vi "phy_packet_decoder.vi"(11 "bits":u8[](array[numeric])) -> (3 "string Array":string[](array[string]))   [LabVIEW 2014]
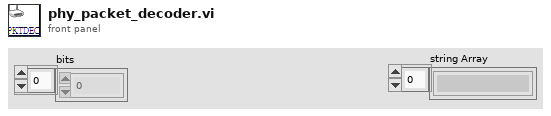
[diagram p1: front panel]
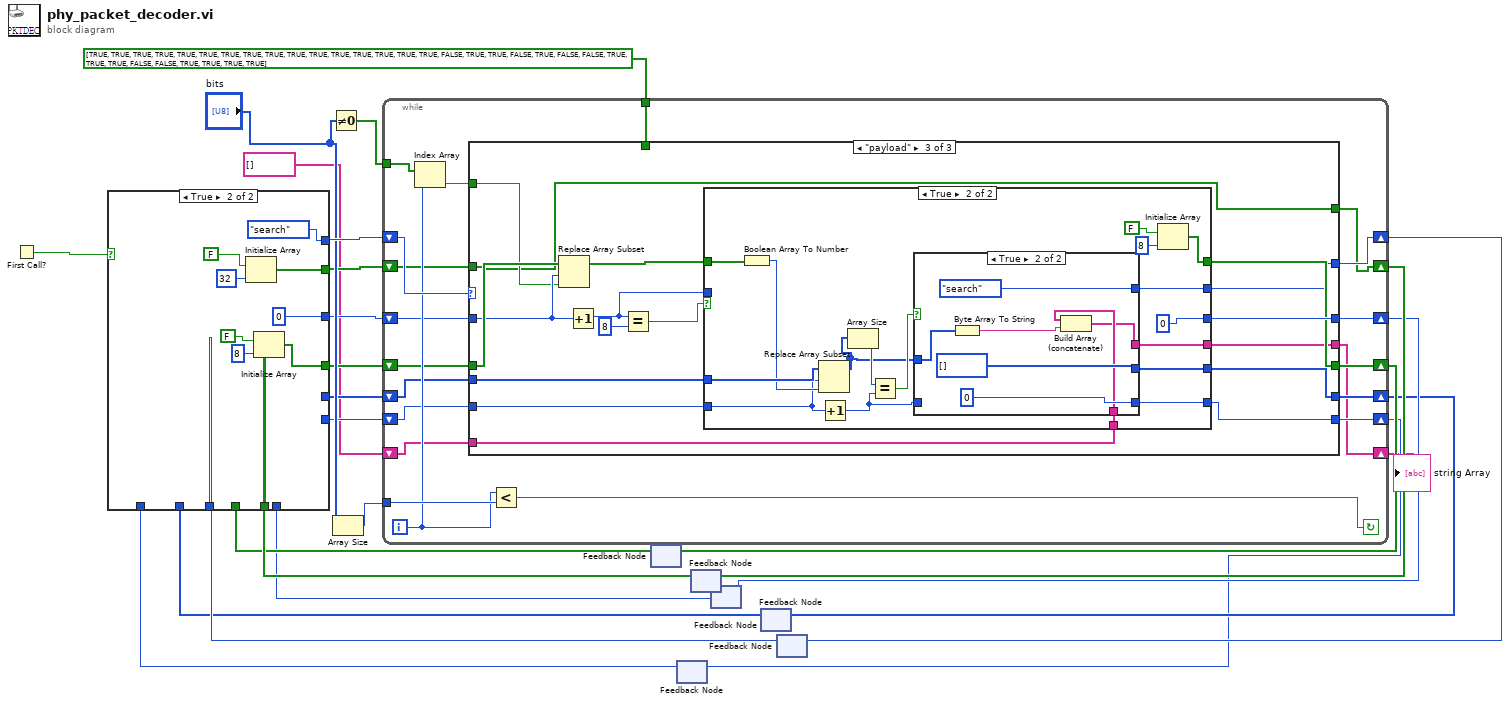
[diagram p0: block diagram]
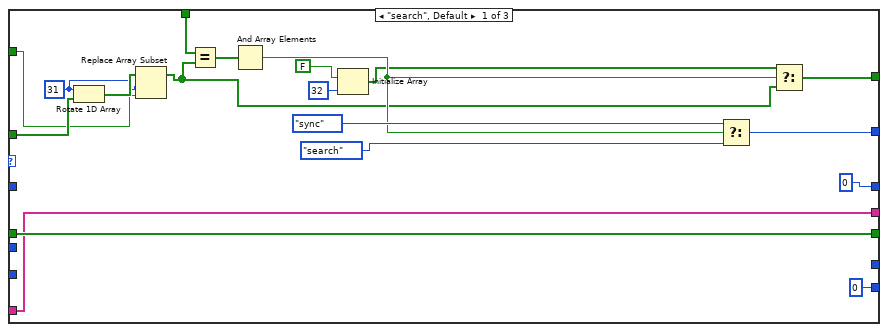
[diagram p3: hidden frame]
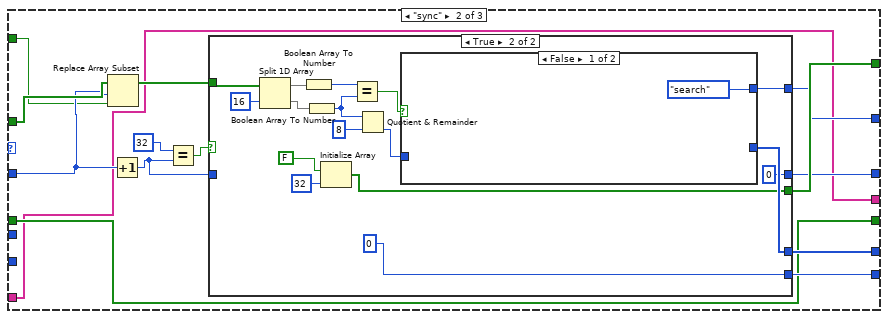
[diagram p4: hidden frame]
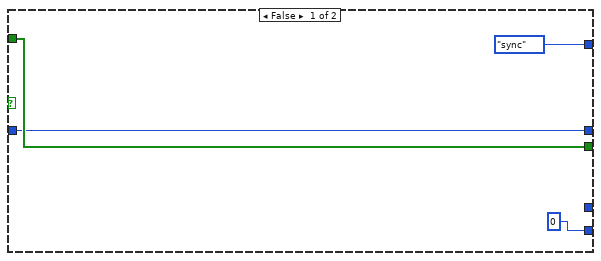
[diagram p5: hidden frame]
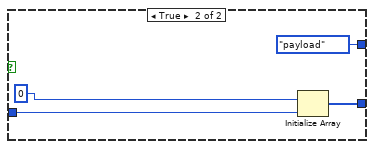
[diagram p6: hidden frame]
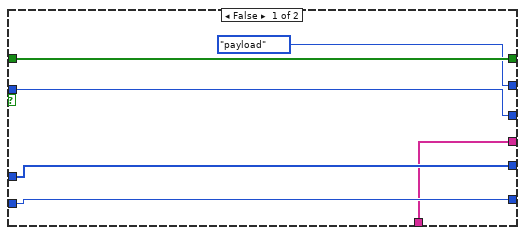
[diagram p7: hidden frame]
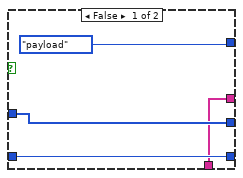
[diagram p8: hidden frame]
diagram:
  n1 = First Call?() -> (First Call?: T/F=w25:bool)
  n2 = Not Equal To 0?(x="bits") -> (x != 0?=w19:bool[])
  n3 = Array Size(array="bits") -> (size(s)=w24:i32)
  n4 = feedback #1() -> (w11:bool[])  [unwired: 1 in]
  n5 = feedback #2() -> (w5:i32)  [unwired: 1 in]
  n6 = feedback #3() -> (w16:bool[])  [unwired: 1 in]
  n7 = feedback #4() -> (w9:i32)  [unwired: 1 in]
  n8 = feedback #5() -> (w7:u8[])  [unwired: 1 in]
  n9 = feedback #6() -> (w21:enum16{"search", "sync", "payload"})  [unwired: 1 in]
  n10 = case shown="True" w25 {
    tunnel: [w31 enum16{"search", "sync", "payload"}."search"] -> w23
    tunnel: w21 -> [w31 _]
    tunnel: [w30 w36] -> w18
    tunnel: w16 -> [w30 _]
    tunnel: [w29 w33] -> w14
    tunnel: [w28 0] -> w13
    tunnel: w11 -> [w29 _]
    tunnel: w9 -> [w28 _]
    tunnel: w7 -> [w26 _]
    tunnel: w5 -> [w27 _]
    tunnel: [w27 _] -> w4
    tunnel: [w26 _] -> w3
    frame False {
    }
    frame True {
      n11 = Initialize Array(FALSE, 32 ("dimension size")) -> (w36:bool[])
      n12 = Initialize Array(FALSE, 8 ("dimension size")) -> (w33:bool[])
    }
  }
  n13 = while {
    shift-right: [w51] -> w22
    shift-left: w23 -> [w57]
    tunnel: w24 -> [w59]
    tunnel: w19 -> [w56]
    shift-right: [w50] -> w17
    shift-left: w18 -> [w53]
    tunnel: bool[] [TRUE, TRUE, TRUE, TRUE, TRUE, TRUE, TRUE, TRUE, TRUE, TRUE, TRUE, TRUE, TRUE, TRUE, TRUE, TRUE, FALSE, TRUE, TRUE, FALSE, TRUE, FALSE, FALSE, TRUE, TRUE, TRUE, FALSE, FALSE, TRUE, TRUE, TRUE, TRUE] ("Boolean array") -> [w52]
    shift-right: [w47] -> w10
    shift-left: w13 -> [w49]
    shift-right: [w46] -> w12
    shift-left: w14 -> [w48]
    shift-right: [w45] -> w8
    shift-left: w3 -> [w42]
    shift-right: [w44] -> w6
    shift-left: w4 -> [w43]
    shift-right: [w40] -> w1
    shift-left: string[] [] -> [w41]
    i -> [w55]
    stop <- w58 continue-if-true
    n14 = Index Array(array=w56, index=w55) -> (element=w54:bool)
    n15 = case shown="\"payload\"" w57 {
      tunnel: w54 -> [w75 w88 w127]
      tunnel: w53 -> [w78 w90 w121]
      tunnel: w52 -> [w74 _ _]
      tunnel: [w70 w83 w120] -> w51
      tunnel: [w64 w84 w121] -> w50
      tunnel: w49 -> [_ w89 w133]
      tunnel: w48 -> [w62 w82 w134]
      tunnel: [0 w80 w130] -> w47
      tunnel: [w62 w82 w122] -> w46
      tunnel: [_ w86 w124] -> w45
      tunnel: [0 w85 w123] -> w44
      tunnel: w43 -> [_ _ w126]
      tunnel: w42 -> [_ _ w125]
      tunnel: w41 -> [w60 w79 w119]
      tunnel: [w60 w79 w118] -> w40
      frame "search", Default {
        w76 = 31 ("n")
        n16 = Rotate 1D Array(1:w78, 2:w76) -> (0:w77:bool[])
        n17 = Replace Array Subset(array=w77, new element=w75, index=w76) -> (w65:bool[])
        n18 = Equal?(x=w74, y=w65) -> (x = y?=w73:bool[])
        n19 = And Array Elements(Boolean array=w73) -> (logical AND=w67:bool)
        n20 = Initialize Array(FALSE, 32 ("dimension size")) -> (w66:bool[])
        n21 = Select(t=enum16{"search", "sync", "payload"}."sync", s=w67, f=enum16{"search", "sync", "payload"}."search") -> (s? t:f=w70:enum16{"search", "sync", "payload"})
        n22 = Select(t=w66, s=w67, f=w65) -> (s? t:f=w64:bool[])
      }
      frame "sync" {
        n23 = Replace Array Subset(array=w90, new element=w88, index=w89) -> (w87:bool[])
        n24 = Increment(x=w89) -> (x+1=w81:i32)
        n25 = Equal?(x=32, y=w81) -> (x = y?=w91:bool)
        n26 = case shown="True" w91 {
          tunnel: w87 -> [w96 w112]
          tunnel: [_ w102] -> w86
          tunnel: [0 0] -> w85
          tunnel: [w96 w99] -> w84
          tunnel: [enum16{"search", "sync", "payload"}."sync" w98] -> w83
          tunnel: w81 -> [w93 _]
          tunnel: [w93 0] -> w80
          frame False {
          }
          frame True {
            n27 = Split 1D Array(array=w112, index=16) -> (first subarray=w110:bool[], second subarray=w109:bool[])
            n28 = Boolean Array To Number(Boolean array=w110) -> (number=w108:u32)
            n29 = Boolean Array To Number(Boolean array=w109) -> (number=w107:u32)
            n30 = Initialize Array(FALSE, 32 ("dimension size")) -> (w99:bool[])
            n31 = Equal?(x=w108, y=w107) -> (x = y?=w104:bool)
            n32 = Quotient & Remainder(x=w107, y=u32 8) -> (floor(x/y)=w103:u32)  [unwired: 1 out]
            n33 = case shown="False" w104 {
              tunnel: w103 -> [_ w116]
              tunnel: [_ w115] -> w102
              tunnel: [enum16{"search", "sync", "payload"}."search" enum16{"search", "sync", "payload"}."payload"] -> w98
              frame False {
              }
              frame True {
                n34 = Initialize Array(u8 0, w116) -> (w115:u8[])
              }
            }
          }
        }
      }
      frame "payload" {
        n35 = Replace Array Subset(array=w134, new element=w127, index=w133) -> (w128:bool[])
        n36 = Increment(x=w133) -> (x+1=w129:i32)
        n37 = Equal?(x=w129, y=8) -> (x = y?=w131:bool)
        n38 = case shown="True" w131 {
          tunnel: [w140 0] -> w130
          tunnel: w129 -> [w140 _]
          tunnel: w128 -> [w137 w156]
          tunnel: w126 -> [w138 w153]
          tunnel: w125 -> [w139 w155]
          tunnel: [w139 w147] -> w124
          tunnel: [w138 w148] -> w123
          tunnel: [w137 w144] -> w122
          tunnel: [enum16{"search", "sync", "payload"}."payload" w143] -> w120
          tunnel: w119 -> [w135 w142]
          tunnel: [w135 w141] -> w118
          frame False {
          }
          frame True {
            n39 = Boolean Array To Number(Boolean array=w156) -> (number=w154:u32)
            n40 = Replace Array Subset(array=w155, new element=w154, index=w153) -> (w150:u8[])
            n41 = Increment(x=w153) -> (x+1=w149:i32)
            n42 = Array Size(array=w150) -> (size(s)=w152:i32)
            n43 = Equal?(x=w152, y=w149) -> (x = y?=w151:bool)
            n44 = case shown="True" w151 {
              tunnel: w150 -> [w160 w166]
              tunnel: w149 -> [w161 _]
              tunnel: [w161 0] -> w148
              tunnel: [w160 u8[] []] -> w147
              tunnel: [enum16{"search", "sync", "payload"}."payload" enum16{"search", "sync", "payload"}."search"] -> w143
              tunnel: w142 -> [w158 w164]
              tunnel: [w158 w163] -> w141
              frame False {
              }
              frame True {
                n45 = Byte Array To String(unsigned byte array=w166) -> (string=w162:string)
                n46 = Build Array (concatenate)(w164, w162) -> (w163:string[])
              }
            }
            n47 = Initialize Array(FALSE, 8 ("dimension size")) -> (w144:bool[])
          }
        }
      }
    }
    n48 = Less?(x=w55, y=w59) -> (x < y?=w58:bool)
  }
  "string Array" <- w1
  n49 = feedback-in #1(w12) -> ()
  n50 = feedback-in #2(w6) -> ()
  n51 = feedback-in #3(w17) -> ()
  n52 = feedback-in #4(w10) -> ()
  n53 = feedback-in #5(w8) -> ()
  n54 = feedback-in #6(w22) -> ()
